vi "Homework 1.vi"() -> ()   [LabVIEW 2020]
panel:
  out "Boolean":bool
  in  "Threhold":dbl
  in  "Slide":dbl(slide) scale=0.0..100.0
  out "Output":string
  in  "Input":string
  out "Slope":dbl
  in  "Y2":dbl
  in  "X2":dbl
  in  "Y1":dbl
  in  "X1":dbl
  # "Slop Calculation"
  # "What do you think\nabout ECE 144?"
  # "Thresholding"
  # "(Notice the output is all UPPERCASE)"
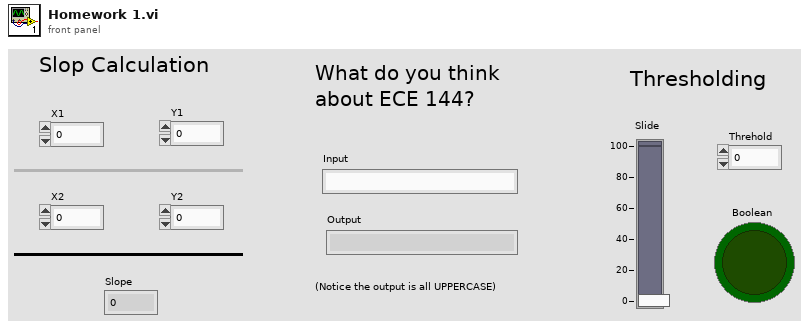
[diagram p1: front panel]
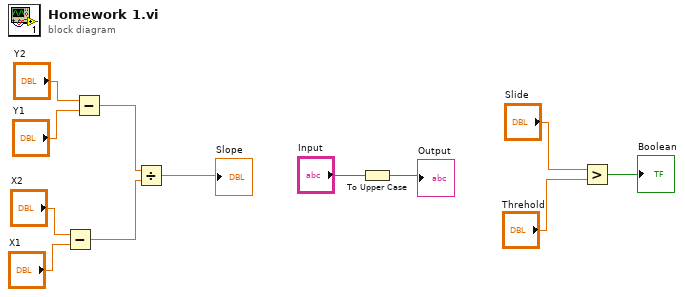
[diagram p0: block diagram]
diagram:
  n1 = Subtract(x="X2", y="X1") -> (x-y=w7:dbl)
  n2 = Subtract(x="Y2", y="Y1") -> (x-y=w8:dbl)
  n3 = Divide(x=w8, y=w7) -> (x/y=→"Slope":dbl)
  n4 = To Upper Case(1:"Input") -> (0:→"Output":string)
  n5 = Greater?(x="Slide", y="Threhold") -> (0:→"Boolean":bool)
